vi "Query System Status.vi"(6 "timeout (ms)":i32=5000, 8 "error in":errorcluster, 9 "Plugin Name":string, 10 "Status":T3 {"Monitor Doubles"."4" format="%#_9g"; "Monitor Doubles"."3" format="%#_9g"; "Monitor Doubles"."2" format="%#_9g"; "Monitor Doubles"."1" format="%#_9g"}, 11 "gRPC ID in":T12) -> (0 "error out":errorcluster, 2 "Clock Conversion Array":T1[](array[typedef]), 3 "gRPC ID out":T12)   [LabVIEW 2021, in "CIFManagerClientWrapper.lvlib"]
uses:
  <vilib>/gRPC/LabVIEW gRPC Library/Shared/grpcId.ctl
  CIFManagerClientWrapper.lvlib
  CIF_Manager_client/CIF_Manager_client.lvlib
  CIF_Manager_client/RPC Messages/cif_manager_PluginName.ctl
  CIF_Manager_client/RPC Messages/cif_plugincore_StatusData_State.ctl
  CIF_Manager_client/RPC Messages/cif_plugincore_TimingStatsBasic.ctl
  CIF_Manager_client/RPC Messages/cif_plugincore_TimingStatistics.ctl
  CIF_Manager_client/RPC Messages/cif_plugincore_FifoStatistics.ctl
  CIF_Manager_client/RPC Messages/cif_plugincore_Error.ctl
  CIF_Manager_client/RPC Messages/cif_plugincore_MonitorDoubles.ctl
  CIF_Manager_client/RPC Messages/cif_plugincore_MonitorU64.ctl
  CIF_Manager_client/RPC Messages/cif_plugincore_MonitorI64.ctl
  CIF_Manager_client/RPC Messages/cif_plugincore_StatusData.ctl
  CIF_Manager_client/RPC Messages/cif_manager_PluginStatus.ctl
  CIFUtilities/CIFClocks/Typedef/Timestamp Pair.ctl
  CIFUtilities/CIFClocks/CIFClocks.lvlib
  CIFUtilities/CIFClocks/Typedef/Clock Conversion.ctl
  <vilib>/gRPC/LabVIEW gRPC Library/grpc-lvsupport-release.lvlib
  CIFCore/Common/Typedef/Plugin State.ctl
  CIFCore/Common/CIFCoreCommon.lvlib
  CIFCore/Common/Typedef/Timing Stats Base.ctl
  CIFCore/Common/Typedef/Timing Statistics.ctl
  CIFCore/Common/Typedef/FIFO Statistics.ctl
  CIFCore/Common/Typedef/Simple Error.ctl
  CIFCore/Common/Typedef/Monitor Doubles.ctl
  CIFCore/Common/Typedef/Monitor U64.ctl
  CIFCore/Common/Typedef/Monitor I64.ctl
  CIFCore/Common/Typedef/Plugin Status.ctl
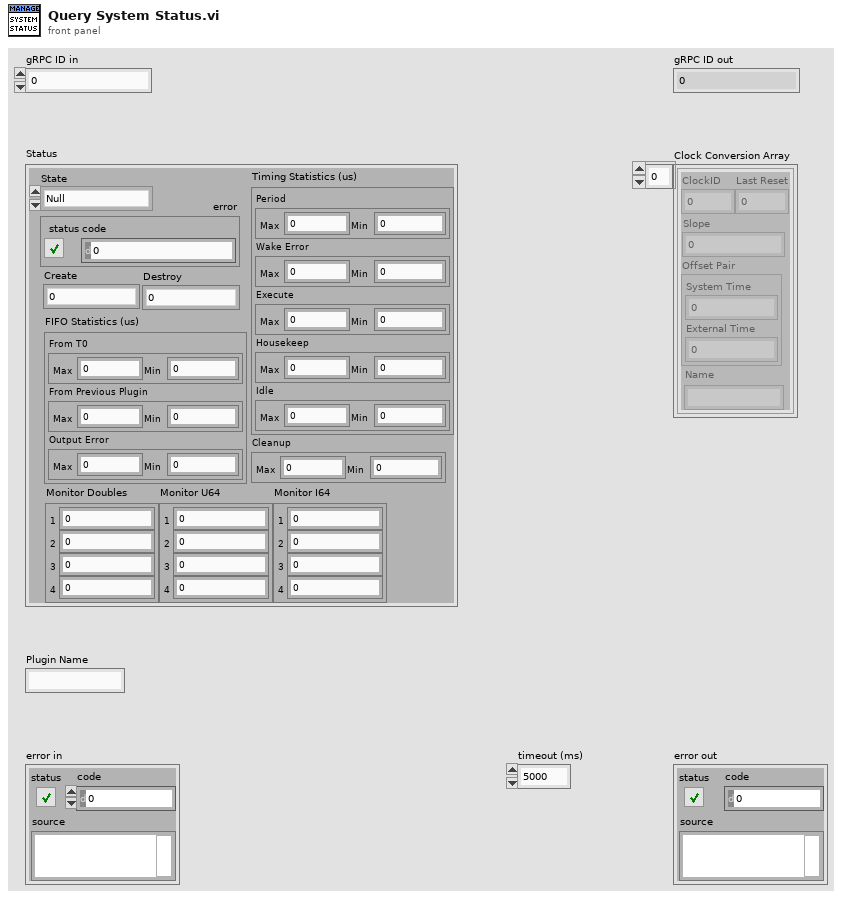
[diagram p1: front panel]
types:
  T1 = typedef "CIFClocks.lvlib/Clock Conversion.ctl" = cluster{"ClockID":u8, "Last Reset":u64, "Offset Pair":T2, "Slope":dbl, "Name":string}
  T2 = typedef "CIFClocks.lvlib/Timestamp Pair.ctl" = cluster{"System Time":i64, "External Time":i64}
  T3 = typedef "CIFCoreCommon.lvlib/Plugin Status.ctl" = cluster{"State":T4, "Timing Statistics (us)":T5, "FIFO Statistics (us)":T7, "error":T8, "Monitor Doubles":T9, "Monitor U64":T10, "Monitor I64":T11, "Cleanup":T6, "Create":i32, "Destroy":i32}
  T4 = typedef "CIFCoreCommon.lvlib/Plugin State.ctl" = enum32{"Null", "Creating", "Listening", "Running", "CleaningUp", "Destroying"}
  T5 = typedef "CIFCoreCommon.lvlib/Timing Statistics.ctl" = cluster{"Period":T6, "Wake Error":T6, "Execute":T6, "Housekeep":T6, "Idle":T6}
  T6 = typedef "CIFCoreCommon.lvlib/Timing Stats Base.ctl" = cluster{"Max":i32, "Min":i32}
  T7 = typedef "CIFCoreCommon.lvlib/FIFO Statistics.ctl" = cluster{"From T0":T6, "From Previous Plugin":T6, "Output Error":T6}
  T8 = typedef "CIFCoreCommon.lvlib/Simple Error.ctl" = cluster{"status":bool, "code":i32}
  T9 = typedef "CIFCoreCommon.lvlib/Monitor Doubles.ctl" = cluster{"1":dbl, "2":dbl, "3":dbl, "4":dbl}
  T10 = typedef "CIFCoreCommon.lvlib/Monitor U64.ctl" = cluster{"1":u64, "2":u64, "3":u64, "4":u64}
  T11 = typedef "CIFCoreCommon.lvlib/Monitor I64.ctl" = cluster{"1":i64, "2":i64, "3":i64, "4":i64}
  T12 = typedef "grpc-lvsupport-release.lvlib/grpcId.ctl" = u64
  T13 = typedef "CIF_Manager_client.lvlib/cif_manager_PluginStatus.ctl" = cluster{"pluginname":T14, "status":T15}
  T14 = typedef "CIF_Manager_client.lvlib/cif_manager_PluginName.ctl" = cluster{"plugin_name":string}
  T15 = typedef "CIF_Manager_client.lvlib/cif_plugincore_StatusData.ctl" = cluster{"state":T16, "timing_statistics":T17, "fifo_statistics":T19, "error":T20, "monitor_doubles":T21, "monitor_u64s":T22, "monitor_i64s":T23}
  T16 = typedef "CIF_Manager_client.lvlib/cif_plugincore_StatusData_State.ctl" = enum32{"NULL", "CREATING", "LISTENING", "RUNNING", "CLEANINGUP", "DESTROYING"}
  T17 = typedef "CIF_Manager_client.lvlib/cif_plugincore_TimingStatistics.ctl" = cluster{"period":T18, "wake_error":T18, "execute":T18, "housekeep":T18, "idle":T18}
  T18 = typedef "CIF_Manager_client.lvlib/cif_plugincore_TimingStatsBasic.ctl" = cluster{"max":i32, "min":i32}
  T19 = typedef "CIF_Manager_client.lvlib/cif_plugincore_FifoStatistics.ctl" = cluster{"from_t0":T18, "from_previous_plugin":T18, "output_error":T18}
  T20 = typedef "CIF_Manager_client.lvlib/cif_plugincore_Error.ctl" = cluster{"status":bool, "code":i32}
  T21 = typedef "CIF_Manager_client.lvlib/cif_plugincore_MonitorDoubles.ctl" = cluster{"double_1":dbl, "double_2":dbl, "double_3":dbl, "double_4":dbl}
  T22 = typedef "CIF_Manager_client.lvlib/cif_plugincore_MonitorU64.ctl" = cluster{"u64_1":u64, "u64_2":u64, "u64_3":u64, "u64_4":u64}
  T23 = typedef "CIF_Manager_client.lvlib/cif_plugincore_MonitorI64.ctl" = cluster{"i64_1":i64, "i64_2":i64, "i64_3":i64, "i64_4":i64}
  T24 = typedef "CIF_Manager_client.lvlib/cif_manager_SystemStatus.ctl" = cluster{"clock_conversion_array":T25}
  T25 = typedef "CIF_Manager_client.lvlib/cif_manager_ClockConversionArray.ctl" = cluster{"clock_conversions":T26[]}
  T26 = typedef "CIF_Manager_client.lvlib/cif_manager_ClockConversion.ctl" = cluster{"clock_id":u32, "last_reset":u64, "slope":dbl, "offset_pair":T27, "clock_name":string}
  T27 = typedef "CIF_Manager_client.lvlib/cif_manager_TimePair.ctl" = cluster{"system_time":i64, "external_time":i64}
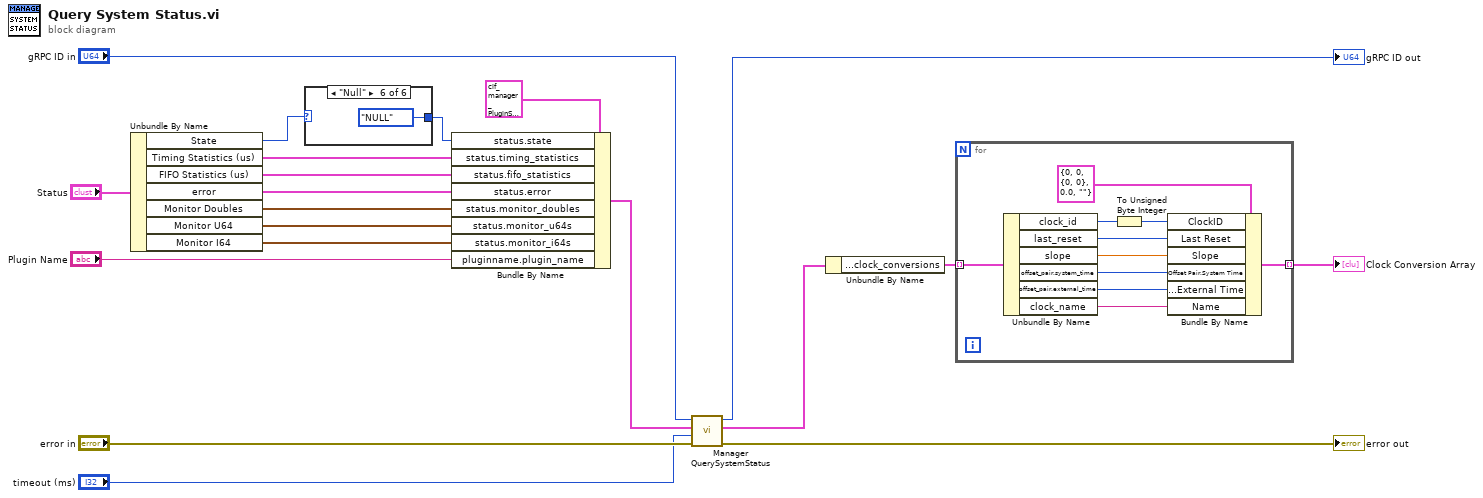
[diagram p0: block diagram]
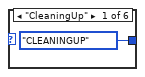
[diagram p2: hidden frame]
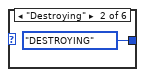
[diagram p3: hidden frame]
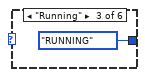
[diagram p4: hidden frame]
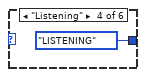
[diagram p5: hidden frame]
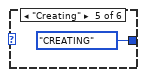
[diagram p6: hidden frame]
diagram:
  n1 = Unbundle By Name("Status") -> ("State"=w7:T4, "Timing Statistics (us)"=w8:T5, "FIFO Statistics (us)"=w9:T7, "error"=w10:T8, "Monitor Doubles"=w11:T9, "Monitor U64"=w12:T10, "Monitor I64"=w13:T11)
  n2 = case shown="\"Null\"" w7 {
    tunnel: [cif_plugincore_StatusData_State."CLEANINGUP" ("status.state") cif_plugincore_StatusData_State."DESTROYING" ("status.state") cif_plugincore_StatusData_State."RUNNING" ("status.state") cif_plugincore_StatusData_State."LISTENING" ("status.state") cif_plugincore_StatusData_State."CREATING" ("status.state") cif_plugincore_StatusData_State."NULL" ("status.state")] -> w6
    frame "CleaningUp" {
    }
    frame "Destroying" {
    }
    frame "Running" {
    }
    frame "Listening" {
    }
    frame "Creating" {
    }
    frame "Null" {
    }
  }
  n3 = Bundle By Name(cluster=T13 {"pluginname"={"plugin_name"=""}, "status"={"state"=enum."NULL", "timing_statistics"={"period"={"max"=0, "min"=0}, "wake_error"={"max"=0, "min"=0}, "execute"={"max"=0, "min"=0}, "housekeep"={"max"=0, "min"=0}, "idle"={"max"=0, "min"=0}}, "fifo_statistics"={"from_t0"={"max"=0, "min"=0}, "from_previous_plugin"={"max"=0, "min"=0}, "output_error"={"max"=0, "min"=0}}, "error"={"status"=FALSE, "code"=0}, "monitor_doubles"={"double_1"=0.0, "double_2"=0.0, "double_3"=0.0, "double_4"=0.0}, "monitor_u64s"={"u64_1"=0, "u64_2"=0, "u64_3"=0, "u64_4"=0}, "monitor_i64s"={"i64_1"=0, "i64_2"=0, "i64_3"=0, "i64_4"=0}}} ("Request Data"), "status.state"=w6, "status.timing_statistics"=w8, "status.fifo_statistics"=w9, "status.error"=w10, "status.monitor_doubles"=w11, "status.monitor_u64s"=w12, "status.monitor_i64s"=w13, "pluginname.plugin_name"="Plugin Name") -> (w4:T13)
  n4 = call "Manager QuerySystemStatus.vi"("error in"="error in", "timeout (ms)"="timeout (ms)", "Request Data"=w4, "gRPC ID"="gRPC ID in") -> ("error out"=→"error out":errorcluster, "Response Data"=w3:T24, "gRPC ID out"=→"gRPC ID out":T12)  [unwired: 5 in]
  n5 = Unbundle By Name(w3) -> ("clock_conversion_array.clock_conversions"=w2:T26[])
  n6 = for {
    tunnel: w2 -> [w36] mode=indexing
    tunnel: [w27] -> w1 mode=indexing
    n7 = Unbundle By Name(w36) -> ("clock_id"=w34:u32, "last_reset"=w31:u64, "slope"=w30:dbl, "offset_pair.system_time"=w29:i64, "offset_pair.external_time"=w28:i64, "clock_name"=w32:string)
    n8 = To Unsigned Byte Integer(number=w34) -> (unsigned 8bit integer=w33:u8)
    n9 = Bundle By Name(cluster=T1 {"ClockID"=0, "Last Reset"=0, "Offset Pair"={"System Time"=0, "External Time"=0}, "Slope"=0.0, "Name"=""} ("Clock Conversion"), "ClockID"=w33, "Last Reset"=w31, "Slope"=w30, "Offset Pair.System Time"=w29, "Offset Pair.External Time"=w28, "Name"=w32) -> (w27:T1)
  }
  "Clock Conversion Array" <- w1
